vi "Truncate According to Map Zoom.vi"(10 "Map reference":refnum<vi>, 11 "data":dbl[][](array[numeric]) format="%.2f") -> (1 "Y Scale.Offset and Multiplier":cluster{"Offset":dbl, "Multiplier":dbl} {"Multiplier" format="%.2f"; "Offset" format="%.2f"}, 2 "X Scale.Offset and Multiplier":cluster{"Offset":dbl, "Multiplier":dbl} {"Multiplier" format="%.2f"; "Offset" format="%.2f"}, 3 "data out":dbl[][](array[numeric]) format="%.2f")   [LabVIEW 2017]
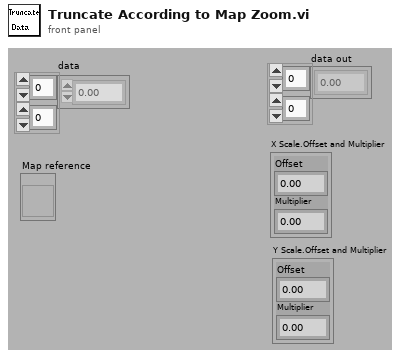
[diagram p1: front panel]
types:
  T1 = typedef "LVOffsetAndMultiplierTypeDef.ctl" = cluster{"Offset":dbl, "Multiplier":dbl}
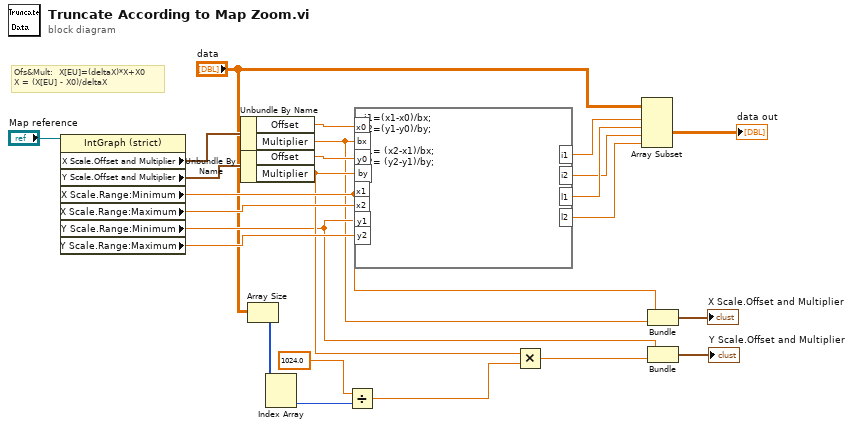
[diagram p0: block diagram]
diagram:
  # "Ofs&Mult:  X[EU]=(deltaX)*X+X0\nX = (X[EU] - X0)/deltaX"
  n1 = property on="Property Node" class="IntGraph (strict)"(reference="Map reference") -> ("X Scale.Offset and Multiplier"=w23:T1, "Y Scale.Offset and Multiplier"=w14:T1, "X Scale.Range:Minimum"=w12:dbl, "X Scale.Range:Maximum"=w20:dbl, "Y Scale.Range:Minimum"=w9:dbl, "Y Scale.Range:Maximum"=w19:dbl)  [unwired: 1 in, 2 out]
  n2 = Unbundle By Name(w23) -> ("Offset"=w22:dbl, "Multiplier"=w1:dbl)
  n3 = Unbundle By Name(w14) -> ("Offset"=w21:dbl, "Multiplier"=w10:dbl)
  n4 = Array Size(array="data") -> (size(s)=w6:i32[])
  n5 = Index Array(array=w6) -> (element #2=w4:i32)  [unwired: 2 in, 1 out]
  n6 = Divide(x=1024.0, y=w4) -> (x/y=w2:dbl)
  n7 = formula code="i1=(x1-x0)/bx;\ni2=(y1-y0)/by;\n\nl1= (x2-x1)/bx;\nl2= (y2-y1)/by;"("x0"=w22, "bx"=w1, "y0"=w21, "by"=w10, "x1"=w12, "x2"=w20, "y1"=w9, "y2"=w19) -> ("i1"=w16:dbl, "i2"=w15:dbl, "l1"=w18:dbl, "l2"=w17:dbl)
  n8 = Multiply(x=w10, y=w2) -> (x*y=w3:dbl)
  n9 = Array Subset(array="data", index (row)=w16, length (row)=w18, index (col)=w15, length (col)=w17) -> (→"data out":dbl[][])
  n10 = Bundle("XScale.Minimum"=w12, "Multiplier"=w1) -> (→"X Scale.Offset and Multiplier":cluster{"XScale.Minimum":dbl, "Multiplier":dbl})  [unwired: 1 in]
  n11 = Bundle("YScale.Minimum"=w9, w3) -> (→"Y Scale.Offset and Multiplier":cluster{"YScale.Minimum":dbl, dbl})  [unwired: 1 in]
